vi "Meter-Gauge Dynamic.vi"(0 "Numeric":dbl format="%#_13g", 1 "Scale.Interpolate Color":bool=TRUE, 5 "Limit Min":dbl, 7 "Limit Max":dbl=100.0, 11 "error in":errorcluster) -> (4 "System Meter":dbl(knob)=21.586596923816817 scale=0.0..100.0, 6 "System Meter 5":dbl(knob)=21.586596923816817 scale=0.0..100.0, 15 "error out":errorcluster)   [LabVIEW 2019]
panel:
  out "Meter Scale.Marker Values":cluster{"Limit":dbl, "Color":u32}[](array[cluster])=[{"Limit"=0.0, "Color"=8191865}, {"Limit"=25.0, "Color"=16448250}, {"Limit"=50.0, "Color"=16448250}, {"Limit"=75.0, "Color"=16448250}, {"Limit"=100.0, "Color"=16448250}]
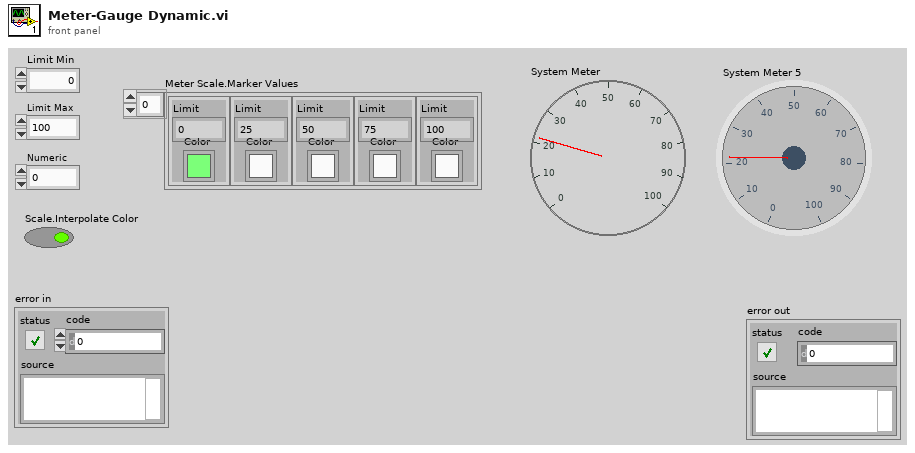
[diagram p1: front panel]
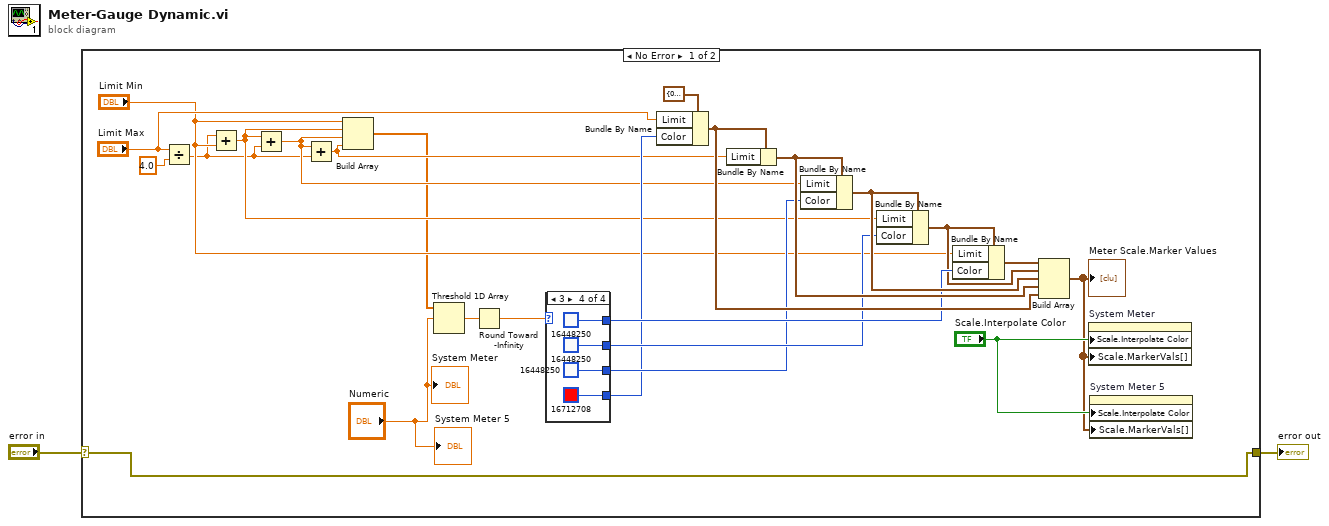
[diagram p0: block diagram]
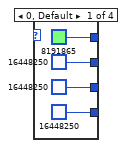
[diagram p2: hidden frame]
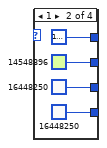
[diagram p3: hidden frame]
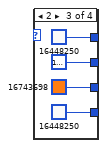
[diagram p4: hidden frame]
diagram:
  n1 = case shown="No Error" "error in" {
    selector: "error in" -> [w3 w43]
    tunnel: [w3 w43] -> w1
    frame No Error {
      n2 = Divide(x="Limit Max", y=4.0) -> (x/y=w7:dbl)
      n3 = Add(x=w7, y="Limit Min") -> (x+y=w9:dbl)
      n4 = Add(x=w9, y=w7) -> (x+y=w8:dbl)
      n5 = Add(x=w8, y=w7) -> (x+y=w6:dbl)
      n6 = Build Array("Limit Min", w9, w8, w6) -> (w4:dbl[])
      n7 = Threshold 1D Array(2:"Numeric", 3:w4) -> (0:w22:dbl)  [unwired: 1 in]
      n8 = Round Toward -Infinity(1:w22) -> (0:w21:dbl)
      n9 = case shown="3" w21 {
        tunnel: [u32 16448250 ("Color 3") u32 16448250 ("Color 3") u32 16448250 ("Color 3") u32 16712708 ("Color 3")] -> w14
        tunnel: [u32 16448250 ("Color 2") u32 14548896 ("Color 2") u32 16777238 ("Color 2") u32 16448250 ("Color 2")] -> w19
        tunnel: [u32 8191865 ("Color 1") u32 16777238 ("Color 1") u32 16448250 ("Color 1") u32 16448250 ("Color 1")] -> w20
        tunnel: [u32 16448250 ("Color 3") u32 16448250 ("Color 3") u32 16743698 ("Color 3") u32 16448250 ("Color 3")] -> w15
        frame 0, Default {
        }
        frame 1 {
        }
        frame 2 {
        }
        frame 3 {
        }
      }
      n10 = Bundle By Name(cluster=cluster{"Limit":dbl, "Color":u32} {"Limit"=0.0, "Color"=16448250}, "Limit"="Limit Max", "Color"=w14) -> (w23:cluster{"Limit":dbl, "Color":u32})
      n11 = Bundle By Name(cluster=w23, "Limit"=w6) -> (w24:cluster{"Limit":dbl, "Color":u32})
      n12 = Bundle By Name(cluster=w24, "Limit"=w8, "Color"=w15) -> (w25:cluster{"Limit":dbl, "Color":u32})
      n13 = Bundle By Name(cluster=w25, "Limit"=w9, "Color"=w19) -> (w17:cluster{"Limit":dbl, "Color":u32})
      n14 = Bundle By Name(cluster=w17, "Limit"="Limit Min", "Color"=w20) -> (w18:cluster{"Limit":dbl, "Color":u32})
      n15 = Build Array(w18, w17, w25, w24, w23) -> (w12:cluster{"Limit":dbl, "Color":u32}[])
      "Meter Scale.Marker Values" <- w12
      n16 = property on="System Meter" class="Knob (strict)"("Scale.Interpolate Color"="Scale.Interpolate Color", "Scale.MarkerVals[]"=w12) -> ()  [unwired: 2 in, 2 out]
      n17 = property on="System Meter 5" class="Knob (strict)"("Scale.Interpolate Color"="Scale.Interpolate Color", "Scale.MarkerVals[]"=w12) -> ()  [unwired: 2 in, 2 out]
      "System Meter" <- "Numeric"
      "System Meter 5" <- "Numeric"
    }
    frame Error {
    }
  }
  "error out" <- w1
